vi "postgres_interval_to_double.vi"(8 "error in (no error)":errorcluster, 11 "postgres_interval":variant) -> (0 "error out":errorcluster, 3 "labview_interval":dbl format="%<%H:%M:%S%3u>t")   [LabVIEW 2015, in "lv-example-postgres.lvlib"]
uses:
  lv-example-postgres.lvlib
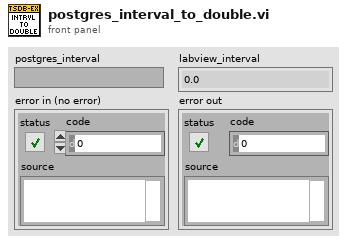
[diagram p1: front panel]
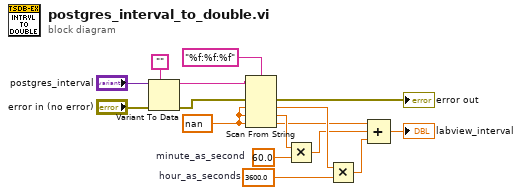
[diagram p0: block diagram]
diagram:
  w14 = nan ("default value 1")
  w13 = 3600.0  # hour_as_seconds
  w12 = 60.0  # minute_as_second
  n1 = Variant To Data(error in="error in (no error)", type="", Variant="postgres_interval") -> (data=w7:string, error out=w4:errorcluster)
  n2 = Scan From String(format string="%f:%f:%f", input string=w7, error in=w4, default 1=w14, default 2=w14, default 3=w14) -> (error out=→"error out":errorcluster, output 1=w10:dbl, output 2=w11:dbl, output 3=w3:dbl)  [unwired: 1 in, 2 out]
  n3 = Multiply(x=w11, y=w12) -> (x*y=w2:dbl)
  n4 = Multiply(x=w10, y=w13) -> (x*y=w1:dbl)
  n5 = Compound Arithmetic op=ADD(w3, w2, w1) -> (→"labview_interval":dbl)
